vi "Test MQTT-4.3.3-1.vi"(8 "error in (no error)":errorcluster, 11 "Connection Config":refnum<class "Connection.lvclass">) -> (0 "error out":errorcluster, 3 "Connection Config dup":refnum<class "Connection.lvclass">)   [LabVIEW 2013]
uses:
  <vilib>/LabVIEW Open Source Project/MQTT Connection/MQTT_Connection/Connection/Connection.lvclass
  <vilib>/LabVIEW Open Source Project/MQTT Control Packets/Control Packets/SUBSCRIBE/Topic Subscription -- cluster.ctl
  <vilib>/LabVIEW Open Source Project/MQTT Control Packets/Control Packets/ControlPacket/QualityOfService -- enum.ctl
  <vilib>/LabVIEW Open Source Project/MQTT Control Packets/Control Packets/ControlPacket/Control Packet Type -- enum.ctl
  <vilib>/LabVIEW Open Source Project/MQTT Control Packets/Control Packets/ControlPacket/ControlPacket.lvclass
  <vilib>/LabVIEW Open Source Project/MQTT Control Packets/Control Packets/ControlPacket/ControlPacket.lvclass/ControlPacket.ctl
  <vilib>/addons/_JKI Toolkits/Caraya/classes/Assert/Assert True.vi
  <vilib>/LabVIEW Open Source Project/MQTT Control Packets/Control Packets/CONNECT/CONNECT.lvclass
  <vilib>/addons/_JKI Toolkits/Caraya/classes/Test/Test.lvclass
  <vilib>/LabVIEW Open Source Project/MQTT Control Packets/Control Packets/DISCONNECT/DISCONNECT.lvclass
  <vilib>/LabVIEW Open Source Project/MQTT Control Packets/Control Packets/SUBSCRIBE/SUBSCRIBE.lvclass
  <vilib>/LabVIEW Open Source Project/MQTT Control Packets/Control Packets/PUBLISH/PUBLISH.lvclass
  <vilib>/addons/_JKI Toolkits/Caraya/classes/Assert/Assert.lvclass
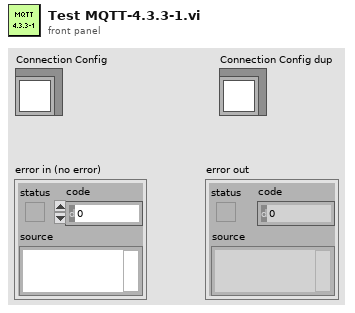
[diagram p1: front panel]
types:
  T1 = typedef "MQTT_Control_Packets.lvlib/ControlPacket.lvclass/Control Packet Type -- enum.ctl" = enum16{"Reserved", "CONNECT", "CONNACK", "PUBLISH", "PUBACK", "PUBREC", "PUBREL", "PUBCOMP", "SUBSCRIBE", "SUBACK", "UNSUBSCRIBE", "UNSUBACK", "PINGREQ", "PINGRESP", "DISCONNECT", "AUTH"}
  T2 = typedef "MQTT_Control_Packets.lvlib/ControlPacket.lvclass/QualityOfService -- enum.ctl" = enum16{"0 (At Most Once)", "1 (At Least Once)", "2 (Exactly Once)"}
  T3 = typedef "MQTT_Control_Packets.lvlib/SUBSCRIBE.lvclass/Topic Subscription -- cluster.ctl" = cluster{"Topic Filter":string, "QoS":T2}
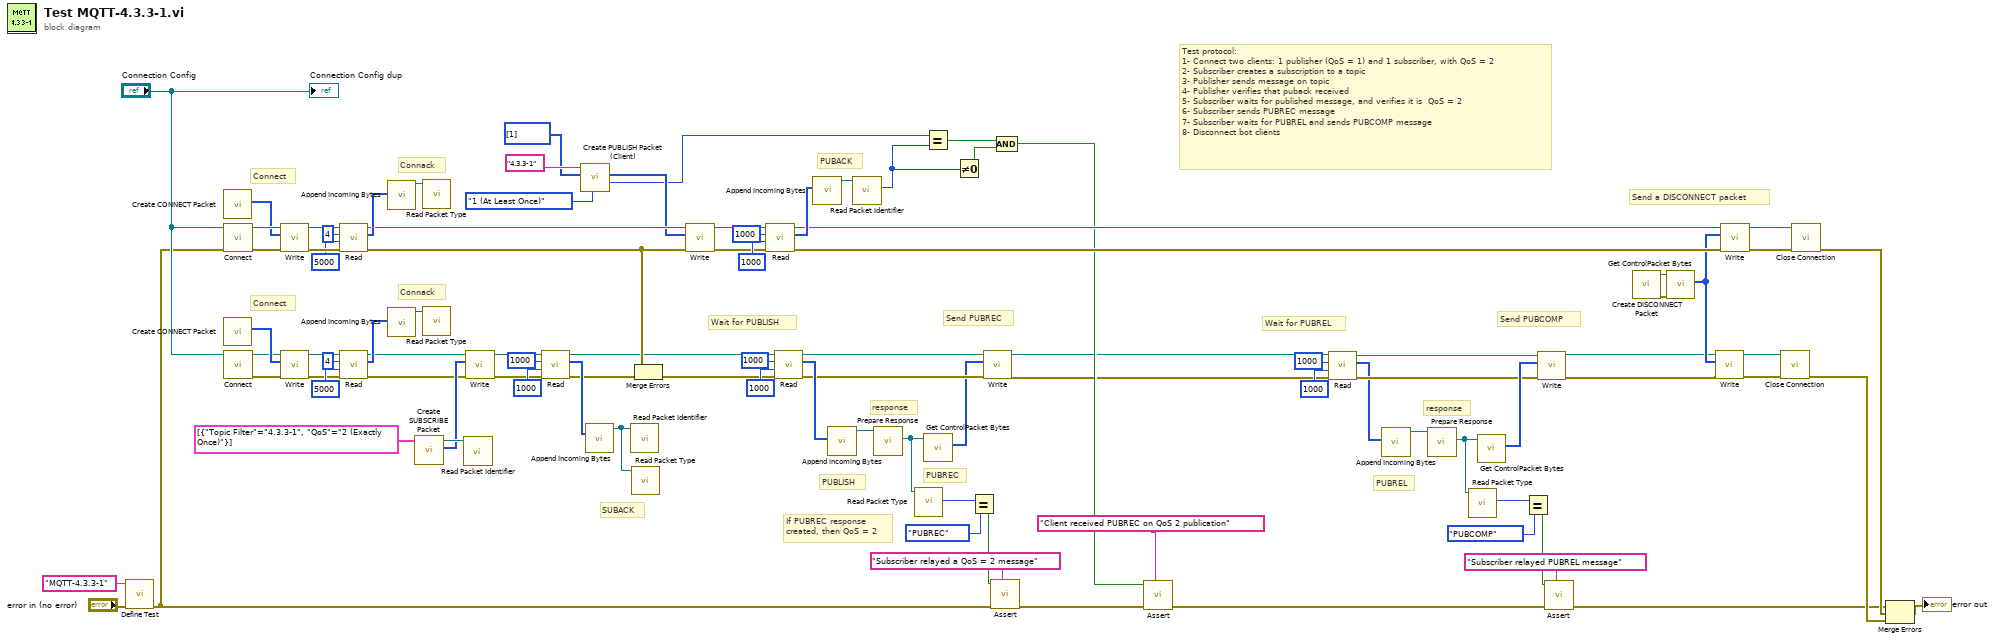
[diagram p0: block diagram]
diagram:
  # "Send PUBCOMP"
  # "response"
  # "PUBREL"
  # "Wait for PUBREL"
  # "Send PUBREC"
  # "If PUBREC response\ncreated, then QoS = 2"
  # "response"
  # "PUBREC"
  # "PUBLISH"
  # "Wait for PUBLISH"
  # "PUBACK"
  # "SUBACK"
  # "Connack"
  # "Connect"
  # "Connack"
  # "Connect"
  # "Test protocol: \n1- Connect two clients: 1 publisher (QoS = 1) and 1 subscriber, with QoS = 2\n2- Subscriber creates a subscription to a topic\n3- Publisher sends message on topic\n4- Publisher verifies that puback received\n5- Subscriber waits for published message, and verifies it is  QoS = 2\n6- Subscriber sends PUBREC message\n7- Subscriber waits for PUBREL and sends PUBCOMP message\n8- Disconnect bot clients"
  # "Send a DISCONNECT packet"
  n1 = call <vilib>:"Define Test.vi"("error in (no error)"="error in (no error)", "Label (VI Title)"="MQTT-4.3.3-1") -> ("error out"=w31:errorcluster)  [unwired: 9 in]
  n2 = call <vilib>:"Create CONNECT Packet.vi"() -> ("Bytes Stream"=w85:u8[])  [unwired: 9 in, 2 out]
  n3 = call <vilib>:"Create CONNECT Packet.vi"() -> ("Bytes Stream"=w79:u8[])  [unwired: 9 in, 2 out]
  n4 = call <vilib>:"Connect.vi"("error in (no error)"=w31, "Connection in"="Connection Config") -> ("error out"=w89:errorcluster, "Connection out"=w88:refnum<class "Connection.lvclass">)  [unwired: 8 in]
  n5 = call <vilib>:"Connect.vi"("Connection in"="Connection Config") -> ("error out"=w76:errorcluster, "Connection out"=w77:refnum<class "Connection.lvclass">)  [unwired: 9 in]
  n6 = call <vilib>:"Write.vi"("error in (no error)"=w89, "Bytes"=w85, "Connection in"=w88) -> ("error out"=w90:errorcluster, "Connection"=w91:refnum<class "Connection.lvclass">)  [unwired: 7 in]
  n7 = call <vilib>:"Write.vi"("error in (no error)"=w76, "Bytes"=w79, "Connection in"=w77) -> ("error out"=w75:errorcluster, "Connection"=w74:refnum<class "Connection.lvclass">)  [unwired: 7 in]
  n8 = call <vilib>:"Read.vi"("error in (no error)"=w90, "timeout (2000 ms)"=5000 ("timeout (1000 ms)"), "bytes to read (100)"=4 ("bytes to read"), "TCPConnection in"=w91) -> ("error out"=w56:errorcluster, "Bytes"=w84:u8[], "TCPConnection out"=w55:refnum<class "Connection.lvclass">)  [unwired: 3 in, 2 out]
  n9 = call <vilib>:"Read.vi"("error in (no error)"=w75, "timeout (2000 ms)"=5000 ("timeout (1000 ms)"), "bytes to read (100)"=4 ("bytes to read"), "TCPConnection in"=w74) -> ("error out"=w67:errorcluster, "Bytes"=w80:u8[], "TCPConnection out"=w69:refnum<class "Connection.lvclass">)  [unwired: 3 in, 2 out]
  n10 = call <vilib>:"Append Incoming Bytes.vi"("Incoming Packets"=w84) -> ("ControlPacket"=w83:refnum<class "ControlPacket.lvclass">)  [unwired: 7 in, 3 out]
  n11 = call <vilib>:"Append Incoming Bytes.vi"("Incoming Packets"=w80) -> ("ControlPacket"=w81:refnum<class "ControlPacket.lvclass">)  [unwired: 7 in, 3 out]
  n12 = call <vilib>:"Create SUBSCRIBE Packet.vi"("Topic Subscriptions"=T3[] [{"Topic Filter"="4.3.3-1", "QoS"=enum."2 (Exactly Once)"}]) -> ("Bytes Stream"=w68:u8[], "SUBSCRIBE out"=w70:refnum<class "SUBSCRIBE.lvclass">)  [unwired: 8 in, 1 out]
  n13 = call <vilib>:"Read Packet Type.vi"("ControlPacket in"=w83) -> ()  [unwired: 9 in, 2 out]
  n14 = call <vilib>:"Read Packet Type.vi"("ControlPacket in"=w81) -> ()  [unwired: 9 in, 2 out]
  n15 = call <vilib>:"Read Packet Identifier.vi"("ControlPacket in"=w70) -> ()  [unwired: 9 in, 2 out]
  n16 = call <vilib>:"Write.vi"("error in (no error)"=w67, "Bytes"=w68, "Connection in"=w69) -> ("error out"=w63:errorcluster, "Connection"=w64:refnum<class "Connection.lvclass">)  [unwired: 7 in]
  n17 = call <vilib>:"Read.vi"("error in (no error)"=w63, "timeout (2000 ms)"=1000 ("timeout (1000 ms)"), "bytes to read (100)"=1000 ("bytes to read"), "TCPConnection in"=w64) -> ("error out"=w60:errorcluster, "Bytes"=w62:u8[], "TCPConnection out"=w42:refnum<class "Connection.lvclass">)  [unwired: 3 in, 2 out]
  n18 = call <vilib>:"Create PUBLISH Packet (Client).vi"("QoS"=QualityOfService_--_enum."1 (At Least Once)", "Payload"=u8[] [1], "Topic Name"="4.3.3-1" ("Topic Filter")) -> ("Packet ID"=w29:u16, "Bytes Stream"=w54:u8[])  [unwired: 5 in, 2 out]
  n19 = call <vilib>:"Append Incoming Bytes.vi"("Incoming Packets"=w62) -> ("ControlPacket"=w61:refnum<class "ControlPacket.lvclass">)  [unwired: 7 in, 3 out]
  n20 = call <vilib>:"Read Packet Identifier.vi"("ControlPacket in"=w61) -> ()  [unwired: 9 in, 2 out]
  n21 = call <vilib>:"Read Packet Type.vi"("ControlPacket in"=w61) -> ()  [unwired: 9 in, 2 out]
  n22 = Merge Errors(w56, w60) -> (w41:errorcluster)
  n23 = call <vilib>:"Write.vi"("error in (no error)"=w56, "Bytes"=w54, "Connection in"=w55) -> ("error out"=w48:errorcluster, "Connection"=w50:refnum<class "Connection.lvclass">)  [unwired: 7 in]
  n24 = call <vilib>:"Read.vi"("error in (no error)"=w48, "timeout (2000 ms)"=1000 ("timeout (1000 ms)"), "bytes to read (100)"=1000 ("bytes to read"), "TCPConnection in"=w50) -> ("error out"=w47:errorcluster, "Bytes"=w53:u8[], "TCPConnection out"=w49:refnum<class "Connection.lvclass">)  [unwired: 3 in, 2 out]
  n25 = call <vilib>:"Read.vi"("error in (no error)"=w41, "timeout (2000 ms)"=1000 ("timeout (1000 ms)"), "bytes to read (100)"=1000 ("bytes to read"), "TCPConnection in"=w42) -> ("error out"=w39:errorcluster, "Bytes"=w45:u8[], "TCPConnection out"=w40:refnum<class "Connection.lvclass">)  [unwired: 3 in, 2 out]
  n26 = call <vilib>:"Append Incoming Bytes.vi"("Incoming Packets"=w53) -> ("ControlPacket"=w46:refnum<class "ControlPacket.lvclass">)  [unwired: 7 in, 3 out]
  n27 = call <vilib>:"Append Incoming Bytes.vi"("Incoming Packets"=w45) -> ("ControlPacket"=w37:refnum<class "ControlPacket.lvclass">)  [unwired: 7 in, 3 out]
  n28 = call <vilib>:"Read Packet Identifier.vi"("ControlPacket in"=w46) -> ("Packet Identifier"=w28:u16)  [unwired: 9 in, 1 out]
  n29 = call-dynamic "Prepare Response.vi"("ControlPacket in"=w37) -> ("ControlPacket response"=w24:refnum<class "ControlPacket.lvclass">)  [unwired: 7 in, 3 out]
  n30 = call <vilib>:"Read Packet Type.vi"("ControlPacket in"=w24) -> ("Control Packet Type"=w23:T1)  [unwired: 9 in, 1 out]
  n31 = Equal?(x=w29, y=w28) -> (x = y?=w26:bool)
  n32 = call <vilib>:"Get ControlPacket Bytes.vi"("ControlPacket"=w24) -> ("Bytes Stream"=w38:u8[])  [unwired: 7 in, 3 out]
  n33 = Not Equal To 0?(x=w28) -> (x != 0?=w27:bool)
  n34 = Equal?(x=w23, y=Control_Packet_Type_--_enum."PUBREC") -> (x = y?=w21:bool)
  n35 = call <vilib>:"Write.vi"("error in (no error)"=w39, "Bytes"=w38, "Connection in"=w40) -> ("error out"=w3:errorcluster, "Connection"=w6:refnum<class "Connection.lvclass">)  [unwired: 7 in]
  n36 = call-poly <vilib>:"Assert.vi"("Label"="Subscriber relayed a QoS = 2 message", "error in (no error)"=w31, "True?"=w21) -> ("error out"=w30:errorcluster)  [unwired: 8 in]
  n37 = Compound Arithmetic op=AND(w26, w27) -> (w25:bool)
  n38 = call-poly <vilib>:"Assert.vi"("Label"="Client received PUBREC on QoS 2 publication", "error in (no error)"=w30, "True?"=w25) -> ("error out"=w2:errorcluster)  [unwired: 8 in]
  n39 = call <vilib>:"Read.vi"("error in (no error)"=w3, "timeout (2000 ms)"=1000 ("timeout (1000 ms)"), "bytes to read (100)"=1000 ("bytes to read"), "TCPConnection in"=w6) -> ("error out"=w11:errorcluster, "Bytes"=w7:u8[], "TCPConnection out"=w10:refnum<class "Connection.lvclass">)  [unwired: 3 in, 2 out]
  n40 = call <vilib>:"Append Incoming Bytes.vi"("Incoming Packets"=w7) -> ("ControlPacket"=w13:refnum<class "ControlPacket.lvclass">)  [unwired: 7 in, 3 out]
  n41 = call-dynamic "Prepare Response.vi"("ControlPacket in"=w13) -> ("ControlPacket response"=w14:refnum<class "ControlPacket.lvclass">)  [unwired: 7 in, 3 out]
  n42 = call <vilib>:"Read Packet Type.vi"("ControlPacket in"=w14) -> ("Control Packet Type"=w15:T1)  [unwired: 9 in, 1 out]
  n43 = call <vilib>:"Get ControlPacket Bytes.vi"("ControlPacket"=w14) -> ("Bytes Stream"=w12:u8[])  [unwired: 7 in, 3 out]
  n44 = Equal?(x=w15, y=Control_Packet_Type_--_enum."PUBCOMP") -> (x = y?=w17:bool)
  n45 = call <vilib>:"Write.vi"("error in (no error)"=w11, "Bytes"=w12, "Connection in"=w10) -> ("error out"=w4:errorcluster, "Connection"=w5:refnum<class "Connection.lvclass">)  [unwired: 7 in]
  n46 = call-poly <vilib>:"Assert.vi"("Label"="Subscriber relayed PUBREL message", "error in (no error)"=w2, "True?"=w17) -> ("error out"=w1:errorcluster)  [unwired: 8 in]
  n47 = call <vilib>:"Create DISCONNECT Packet.vi"() -> ("error out"=w94:errorcluster, "DISCONNECT"=w93:refnum<class "DISCONNECT.lvclass">)  [unwired: 9 in, 1 out]
  n48 = call <vilib>:"Get ControlPacket Bytes.vi"("error in (no error)"=w94, "ControlPacket"=w93) -> ("Bytes Stream"=w35:u8[])  [unwired: 6 in, 3 out]
  n49 = call <vilib>:"Write.vi"("error in (no error)"=w4, "Bytes"=w35, "Connection in"=w5) -> ("error out"=w33:errorcluster, "Connection"=w34:refnum<class "Connection.lvclass">)  [unwired: 7 in]
  n50 = call <vilib>:"Write.vi"("error in (no error)"=w47, "Bytes"=w35, "Connection in"=w49) -> ("error out"=w36:errorcluster, "Connection"=w87:refnum<class "Connection.lvclass">)  [unwired: 7 in]
  n51 = call <vilib>:"Close Connection.vi"("error in (no error)"=w33, "Connection in"=w34) -> ("error out"=w32:errorcluster)  [unwired: 8 in, 1 out]
  n52 = call <vilib>:"Close Connection.vi"("error in (no error)"=w36, "Connection in"=w87) -> ("error out"=w82:errorcluster)  [unwired: 8 in, 1 out]
  n53 = Merge Errors(w1, w82, w32) -> (→"error out":errorcluster)
  "Connection Config dup" <- "Connection Config"
